vi "proc_write_stdin.vi"(8 "error in":errorcluster, 10 "write buffer":string, 11 "process instance handle in":u32[](array[numeric])) -> (0 "error out":errorcluster, 2 "bytes written":i32, 3 "process instance handle out":u32[](array[numeric]))   [LabVIEW 2012]
doc: "Writes string to stdin pipe of the process instance."
panel:
  in  "written mem":i32
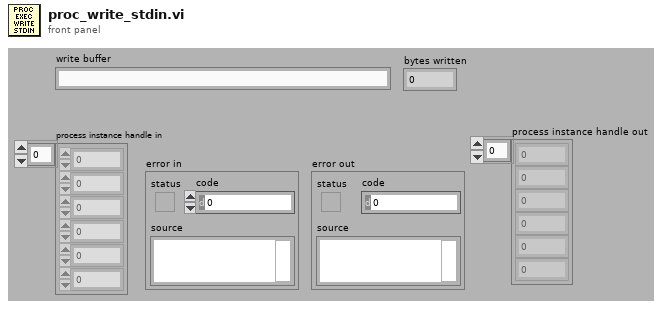
[diagram p1: front panel]
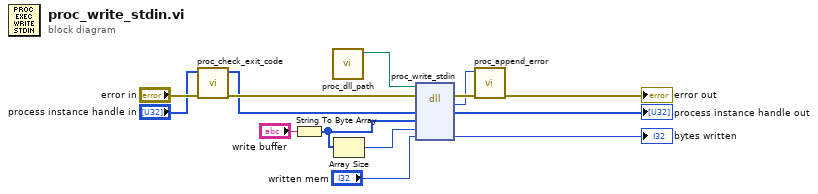
[diagram p0: block diagram]
diagram:
  n1 = call "proc_check_exit_code.vi"("error in"="error in", "instance handle in"="process instance handle in") -> ("error out"=w11:errorcluster, "instance handle out"=w10:u32[])  [unwired: 5 in, 3 out]
  n2 = String To Byte Array(string="write buffer") -> (unsigned byte array=w4:u8[])
  n3 = call "proc_dll_path.vi"() -> ("path out"=w7:path)  [unwired: 10 in, 1 out]
  n4 = Array Size(array=w4) -> (size(s)=w3:i32)
  n5 = dll-call lib="lv_proc.dll" fn="proc_write_stdin"(path in=w7, error in=w11, "proc"=w10, "buffer"=w4, "size"=w3, "written"="written mem") -> (error out=w2:errorcluster, "error"=w1:i32, "proc"=→"process instance handle out":u32[], "written"=→"bytes written":i32)  [unwired: 3 in, 1 out]
  n6 = call "proc_append_error.vi"("error in"=w2, "code in"=w1) -> ("error out"=→"error out":errorcluster)  [unwired: 8 in, 1 out]
